vi "ConnectionTypeToString.vi"(1 "Connection Type":T1) -> (0 "String":string)   [LabVIEW 2010]
uses:
  <vilib>/NXT/NXT Controls/ConnectionType.ctl
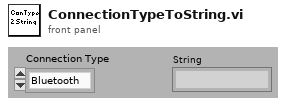
[diagram p1: front panel]
types:
  T1 = typedef "ConnectionType.ctl" = enum16{"Bluetooth", "USB"}
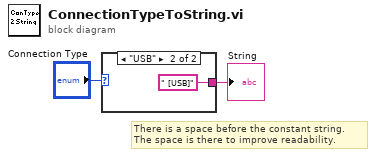
[diagram p0: block diagram]
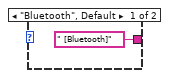
[diagram p2: hidden frame]
diagram:
  # "There is a space before the constant string.\nThe space is there to improve readability."
  n1 = case shown="\"USB\"" "Connection Type" {
    tunnel: [" [Bluetooth]" " [USB]"] -> w2
    frame "Bluetooth", Default {
    }
    frame "USB" {
    }
  }
  "String" <- w2
